vi "KinectCode.vi"() -> ()   [LabVIEW 2013]
uses:
  <vilib>/addons/Kinect/Skeleton Vertex Index.ctl
panel:
  out "Hot? 2":bool
  out "Distance":sgl
  in  "DistanceVariable":sgl
  out "Hot?":bool
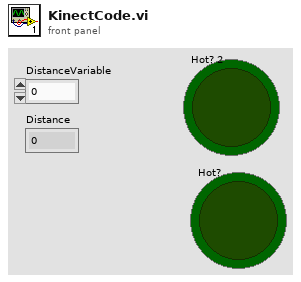
[diagram p1: front panel]
types:
  T1 = typedef "Skeleton Vertex Index.ctl" = i32
  T2 = typedef "SkeletonVertexTrackState.ctl" = enum32{"NotTracked", "Inferred", "Tracked"}
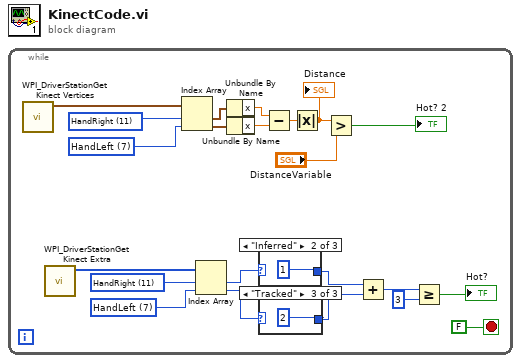
[diagram p0: block diagram]
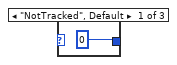
[diagram p2: hidden frame]
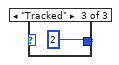
[diagram p3: hidden frame]
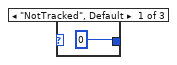
[diagram p4: hidden frame]
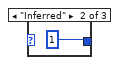
[diagram p5: hidden frame]
diagram:
  n1 = while {
    stop <- FALSE stop-if-true
    w9 = T1 7 items=["HipCenter", "Spine", "ShoulderCenter", "Head", "ShoulderLeft", "ElbowLeft", "WristLeft", "HandLeft", "ShoulderRight", "ElbowRight", "WristRight", "HandRight", "HipLeft", "KneeLeft", "AnkleLeft", "FootLeft", "HipRight", "KneeRight", "AnkleRight", "FootRight"] ("Skeleton Joints")
    w10 = T1 11 items=["HipCenter", "Spine", "ShoulderCenter", "Head", "ShoulderLeft", "ElbowLeft", "WristLeft", "HandLeft", "ShoulderRight", "ElbowRight", "WristRight", "HandRight", "HipLeft", "KneeLeft", "AnkleLeft", "FootLeft", "HipRight", "KneeRight", "AnkleRight", "FootRight"] ("Skeleton Joints")
    w20 = T1 7 items=["HipCenter", "Spine", "ShoulderCenter", "Head", "ShoulderLeft", "ElbowLeft", "WristLeft", "HandLeft", "ShoulderRight", "ElbowRight", "WristRight", "HandRight", "HipLeft", "KneeLeft", "AnkleLeft", "FootLeft", "HipRight", "KneeRight", "AnkleRight", "FootRight"] ("Skeleton Joints")
    w21 = T1 11 items=["HipCenter", "Spine", "ShoulderCenter", "Head", "ShoulderLeft", "ElbowLeft", "WristLeft", "HandLeft", "ShoulderRight", "ElbowRight", "WristRight", "HandRight", "HipLeft", "KneeLeft", "AnkleLeft", "FootLeft", "HipRight", "KneeRight", "AnkleRight", "FootRight"] ("Skeleton Joints")
    n2 = call <vilib>:"WPI_DriverStationGet Kinect Vertices.vi"() -> ("Skeleton Vertices"=w11:cluster{"x":sgl, "y":sgl, "z":sgl}[])  [unwired: 10 in, 1 out]
    n3 = call <vilib>:"WPI_DriverStationGet Kinect Extra.vi"() -> ("Skeleton Tracking State"=w22:T2[])  [unwired: 7 in, 4 out]
    n4 = Index Array(array=w11, index #1=w10, index #2=w9) -> (element #1=w8:cluster{"x":sgl, "y":sgl, "z":sgl}, element #2=w7:cluster{"x":sgl, "y":sgl, "z":sgl})
    n5 = Index Array(array=w22, index #1=w21, index #2=w20) -> (element #1=w17:T2, element #2=w18:T2)
    n6 = Unbundle By Name(w8) -> ("x"=w5:sgl)
    n7 = Unbundle By Name(w7) -> ("x"=w6:sgl)
    n8 = case shown="\"Inferred\"" w17 {
      tunnel: [0 1 2] -> w16
      frame "NotTracked", Default {
      }
      frame "Inferred" {
      }
      frame "Tracked" {
      }
    }
    n9 = case shown="\"Tracked\"" w18 {
      tunnel: [0 1 2] -> w15
      frame "NotTracked", Default {
      }
      frame "Inferred" {
      }
      frame "Tracked" {
      }
    }
    n10 = Subtract(x=w5, y=w6) -> (x-y=w4:sgl)
    n11 = Absolute Value(x=w4) -> (abs(x)=w3:sgl)
    "Distance" <- w3
    n12 = Greater?(x=w3, y="DistanceVariable") -> (0:→"Hot? 2":bool)
    n13 = Add(x=w16, y=w15) -> (x+y=w14:i32)
    n14 = Greater Or Equal?(x=w14, y=3) -> (x >= y?=→"Hot?":bool)
  }
